vi "SetLimiterPopUp.vi"(8 "error in":T7) -> (0 "error out":T7)   [LabVIEW 2016]
doc: "This VI will show its front panel when it is called. You can now enter the desired variables into the input cluster. If you want to set the entered values, press the \"set values\" button below the clusters. The values will be set and the pop-up window will be closed afterwards. The input cluster contains the following variables:\n- Mode (integer) [0-2 -- Spectroscopy1-3]\n- Active (integer) [0 -- off; 1 -- on]\n- Source (integer) [0-5 -- ADC1-6; 6 -- SPM Z out; 7 -- SPM Z out inv; 8 -- AFM Signal; 9 -- AFM df; 10 -- AFM Aexc; 11 -- AFM Aosc; 12 -- AFM Phase; 13 -- LockIn Ampl; 14 -- LockIn Phase]\n- Sign (integer) [0 -- Source > Value; 1-- Source < Value]"
uses:
  Controls/Error_Out.ctl
  Controls/Limiter_Parameters.ctl
  Controls/Limiter-Active_Selection.ctl
  Controls/Limiter-Source_Selection.ctl
  Controls/Limiter-Sign_Selection.ctl
  Controls/Spectroscopy-loop_Selection.ctl
  Controls/Spectroscopy-Mode_Selection.ctl
panel:
  in  "Set values":bool
  out "Output Cluster":T1={"Limit"=FALSE, "Source"=-2147483648, "Value a.u."=-inf, "Sign"=-2147483648, "Loop"=FALSE, "Mode"=0} {"Mode" items=["Spectroscopy 1", "Spectroscopy 2", "Spectroscopy 3", "Calibration"]; "Sign" items=["[read only]"=-2147483648, "Source > Value"=0, "Source < Value"=1]; "Source" items=["[read only]"=-2147483648, "ADC 1"=0, "ADC 2"=1, "ADC 3"=2, "ADC 4"=3, "ADC 5"=4, "ADC 6"=5, "HF 1 Out"=7, "HF 1 df"=8, "SPM Z Out"=9, "HF 1"=12, "HF 1 Ampl"=13, "HF 1 Phase"=14, "LF LockIn Ampl"=16, "LF LockIn Phase"=17, "SPM Z Out inv"=18, "Counter"=23, "Crosslink 1"=29, "Crosslink 2"=30, "Pos X"=31, "Pos Y"=32]}
  in  "Limiter Cluster":T1={"Limit"=FALSE, "Source"=-2147483648, "Value a.u."=-inf, "Sign"=-2147483648, "Loop"=FALSE, "Mode"=0} {"Mode" items=["Spectroscopy 1", "Spectroscopy 2", "Spectroscopy 3", "Calibration"]; "Sign" items=["[read only]"=-2147483648, "Source > Value"=0, "Source < Value"=1]; "Source" items=["[read only]"=-2147483648, "ADC 1"=0, "ADC 2"=1, "ADC 3"=2, "ADC 4"=3, "ADC 5"=4, "ADC 6"=5, "HF 1 Out"=7, "HF 1 df"=8, "SPM Z Out"=9, "HF 1"=12, "HF 1 Ampl"=13, "HF 1 Phase"=14, "LF LockIn Ampl"=16, "LF LockIn Phase"=17, "SPM Z Out inv"=18, "Counter"=23, "Crosslink 1"=29, "Crosslink 2"=30, "Pos X"=31, "Pos Y"=32]}
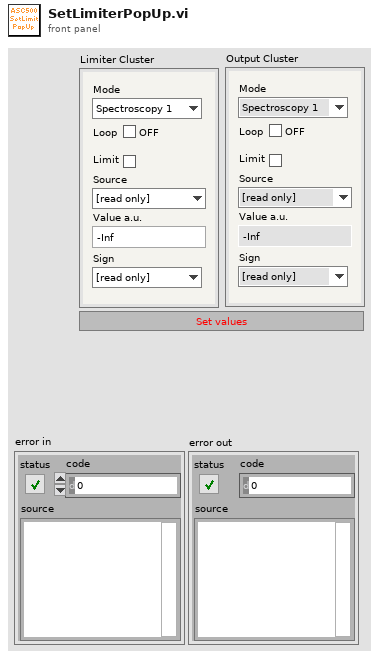
[diagram p1: front panel]
types:
  T1 = typedef "Limiter_Parameters.ctl" = cluster{"Limit":T2, "Source":T3, "Value a.u.":sgl, "Sign":T4, "Loop":T5, "Mode":T6}
  T2 = typedef "Limiter-Active_Selection.ctl" = bool
  T3 = typedef "Limiter-Source_Selection.ctl" = i32
  T4 = typedef "Limiter-Sign_Selection.ctl" = i32
  T5 = typedef "Spectroscopy-loop_Selection.ctl" = bool
  T6 = typedef "Spectroscopy-Mode_Selection.ctl" = u16
  T7 = typedef "Error_Out.ctl" = errorcluster
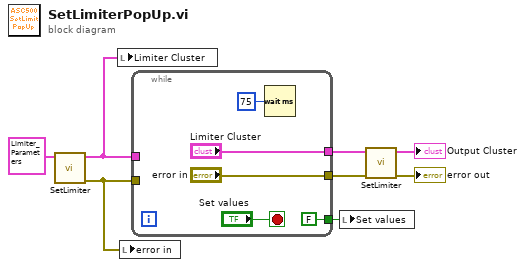
[diagram p0: block diagram]
diagram:
  n1 = call "SetLimiter.vi"("Limiter Cluster"=T1 {"Limit"=FALSE, "Source"=-2147483648, "Value a.u."=-inf, "Sign"=-2147483648, "Loop"=FALSE, "Mode"=0}) -> ("error out"=w2:T7, "Output Cluster"=w3:T1)  [unwired: 9 in]
  n2 = local write "Limiter Cluster"(w3) -> ()
  n3 = local write "error in"(w2) -> ()
  n4 = while {
    tunnel: ["error in"] -> w8
    tunnel: ["Limiter Cluster"] -> w6
    tunnel: [FALSE] -> w4
    tunnel: w2 -> [_]
    tunnel: w3 -> [_]
    stop <- "Set values" stop-if-true
    n5 = Wait (ms)(milliseconds to wait=u32 75) -> ()  [unwired: 1 out]
  }
  n6 = local write "Set values"(w4) -> ()
  n7 = call "SetLimiter.vi"("error in"=w8, "Limiter Cluster"=w6) -> ("error out"=→"error out":T7, "Output Cluster"=→"Output Cluster":T1)  [unwired: 8 in]
